vi "Fpga-6592-Top-Level.vi"() -> ()   [LabVIEW 2017]
uses:
  <vilib>/Platform/TimedLoop/XDataNode/timing_clust.ctl
  <vilib>/Platform/TimedLoop/XDataNode/nitl_modes.ctl
  <vilib>/Platform/TimedLoop/XDataNode/wakeup.ctl
  <vilib>/rvi/Emulation/niFpgaSctlEmulationGetInTimedLoop.vi
  <vilib>/rvi/Emulation/niFpgaEmulationReportErrorSimple.vi
  <vilib>/rvi/Emulation/niFpgaGetClockAttributes.vi
  <vilib>/rvi/Emulation/niFpgaCriticalErrorInLSC.vi
  <vilib>/rvi/eio/common/nirviEmuTemplateMethod_errors.vi
  <vilib>/rvi/interface/RandomDataEmulation/niFpgaRandomDataHandleErrors.vi
  <vilib>/Platform/TimedLoop/XDataNode/XDataNode.xnode
  <vilib>/eio/EIONode/EIONode.xnode
  <vilib>/rvi/DataTransferAndStorage/Container/XNode/niFpgaContainer.xnode
  <vilib>/rvi/interface/RandomDataEmulation/nirviRandomDataFpgaReadWriteTemplate.vi
  <vilib>/Platform/TimedLoop/XDataNode/XDNodeRunTimeDep.lvlib
panel:
  out "BUS_address":u32
  out "write_data":u32
  out "addr_strobe_count":u16
  out "write_strobe_count":u16
  out "read_strobe_count":u16
  in  "d_mcs_i\\IO_BUS_read_data":u32
  in  "Pulse":bool
  in  "d_mcs_i\\INTC_Interrupt":fxp<+,4,4>
  out "d_mcs_i\\gpio3_rtl_tri_o":u32
  in  "Write Interrupt":bool
  out "d_mcs_i\\gpio2_rtl_tri_o":u32
  out "d_mcs_i\\gpio1_rtl_tri_o":u32
  in  "d_mcs_i\\gpio_rtl_tri_i":u32
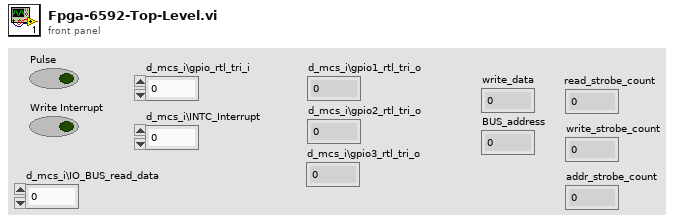
[diagram p1: front panel]
types:
  T1 = typedef "XDNodeRunTimeDep.lvlib/timing_clust.ctl" = cluster{"Expected End [f-1]":u64, "Actual End [f-1]":u64, "Finished Late? [f-1]":bool, "Expected End [i-1]":u64, "Actual End [i-1]":u64, "Finished Late? [i-1]":bool, "Expected Start [i]":u64, "Actual Start [i]":u64, "Expected Start [f]":u64, "Actual Start [f]":u64, "Source Name":string, "Structure Name":string, "Period":i64, "Deadline":i64, "Offset":i64, "Start":i64, "Priority":i32, "Timeout":i32, "Mode":T2, "Wakeup Reason":T3, "Error":errorcluster, "Source Type":string, "Secondary Source Type":string, "Global End Time":u64, "Global Start Time":u64, "Frame Duration":u64, "Iteration Duration":u64, "Assigned CPU":i32, "I/O Scan Engine Mode":u32}
  T2 = typedef "XDNodeRunTimeDep.lvlib/nitl_modes.ctl" = enum32{"No Change", "Process missed periods, maintain original phase", "Discard missed periods, maintain original phase", "Process missed periods, ignore original phase", "Discard missed periods, ignore original phase"}
  T3 = typedef "XDNodeRunTimeDep.lvlib/wakeup.ctl" = enum32{"Normal", "Aborted", "Asynchronous wakeup", "Timing source error", "Timed loop error", "Timeout"}
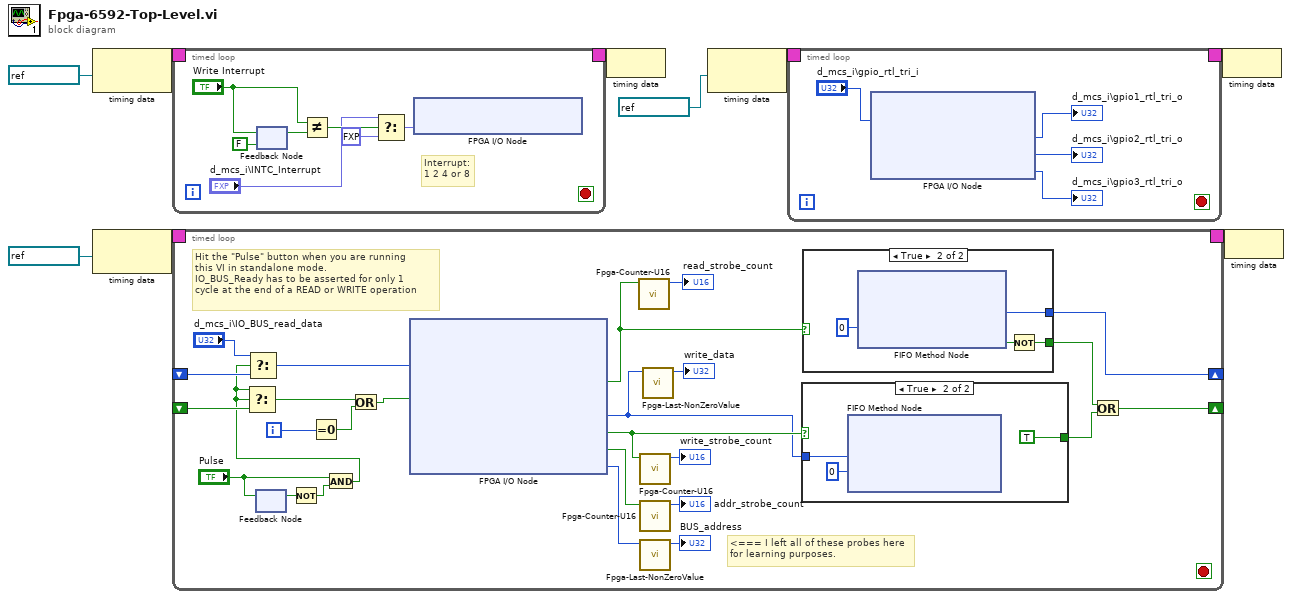
[diagram p0: block diagram]
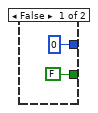
[diagram p2: hidden frame]
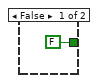
[diagram p3: hidden frame]
diagram:
  n1 = node-c288(refnum<k21> "100MHz" ("Source Name")) -> (w6:T1)
  n2 = node-c288(refnum<k21> "100MHz" ("Source Name")) -> (w9:T1)
  n3 = timed-loop {
    timing: w6 -> [_]
    timing-out: [_] -> w5
    stop <- _ stop-if-true
    # "Interrupt:\n1 2 4 or 8"
    n4 = feedback-in #1("Write Interrupt") -> ()
    n5 = feedback #1(FALSE ("Write Interrupt")) -> (w16:bool)
    n6 = Not Equal?(x="Write Interrupt", y=w16) -> (x != y?=w13:bool)
    n7 = Select(t="d_mcs_i\\INTC_Interrupt", s=w13, f=fxp<+,4,4> 0.0) -> (s? t:f=w11:fxp<+,4,4>)
    n8 = xnode "FPGA I/O Node"("d_mcs_i\\INTC_Interrupt"=w11) -> ()  [unwired: 1 in, 1 out]
  }
  n9 = timed-loop {
    timing: w9 -> [_]
    timing-out: [_] -> w8
    shift-right: [w34] -> _
    shift-left: _ -> [w38]
    shift-right: [w42] -> _
    shift-left: _ -> [w36]
    i -> [w33]
    stop <- _ stop-if-true
    # "Hit the \"Pulse\" button when you are running\nthis VI in standalone mode.\nIO_BUS_Ready has to be asserted for only 1\ncycle at the end of a READ or WRITE operation"
    # "<=== I left all of these probes here\nfor learning purposes."
    n10 = feedback #2() -> (w41:bool)  [unwired: 1 in]
    n11 = feedback-in #2("Pulse") -> ()
    n12 = Not(x=w41) -> (.not. x?=w40:bool)
    n13 = Equal To 0?(x=w33) -> (x = 0?=w19:bool)
    n14 = And(x="Pulse", y=w40) -> (x .and. y?=w22:bool)
    n15 = Select(t=w22, s=w22, f=w38) -> (s? t:f=w21:bool)
    n16 = Select(t="d_mcs_i\\IO_BUS_read_data", s=w22, f=w36) -> (s? t:f=w35:u32)
    n17 = Or(x=w21, y=w19) -> (x .or. y?=w20:bool)
    n18 = xnode "FPGA I/O Node"("d_mcs_i\\IO_BUS_read_data"=w35, "d_mcs_i\\IO_BUS_ready"=w20) -> ("d_mcs_i\\IO_BUS_read_strobe"=w31:bool, "d_mcs_i\\IO_BUS_write_data"=w26:u32, "d_mcs_i\\IO_BUS_write_strobe"=w30:bool, "d_mcs_i\\IO_BUS_addr_strobe"=w27:bool, "d_mcs_i\\IO_BUS_address"=w23:u32)  [unwired: 8 in, 9 out]
    n19 = call "Fpga-Counter-U16.vi"("d_mcs_i\\IO_BUS_read_strobe"=w31) -> ("Numeric"=→"read_strobe_count":u16)  [unwired: 10 in]
    n20 = call "Fpga-Counter-U16.vi"("d_mcs_i\\IO_BUS_read_strobe"=w30) -> ("Numeric"=→"write_strobe_count":u16)  [unwired: 10 in]
    n21 = call "Fpga-Counter-U16.vi"("d_mcs_i\\IO_BUS_read_strobe"=w27) -> ("Numeric"=→"addr_strobe_count":u16)  [unwired: 10 in]
    n22 = call "Fpga-Last-NonZeroValue.vi"("d_mcs_i\\IO_BUS_write_data in"=w23) -> ("d_mcs_i\\IO_BUS_write_data out"=→"BUS_address":u32)  [unwired: 10 in]
    n23 = call "Fpga-Last-NonZeroValue.vi"("d_mcs_i\\IO_BUS_write_data in"=w26) -> ("d_mcs_i\\IO_BUS_write_data out"=→"write_data":u32)  [unwired: 10 in]
    n24 = case shown="True" w30 {
      tunnel: w26 -> [_ w53]
      tunnel: [FALSE TRUE] -> w44
      frame False {
      }
      frame True {
        n25 = xnode ("FIFO Method Node")("Element"=w53, "Timeout"=0) -> ()  [unwired: 1 in, 2 out]
      }
    }
    n26 = case shown="True" w31 {
      tunnel: [FALSE w47] -> w43
      tunnel: [u32 0 ("Element") w48] -> w42
      frame False {
      }
      frame True {
        n27 = xnode ("FIFO Method Node")("Timeout"=0) -> ("Element"=w48:u32, "Timed Out?"=w49:bool)  [unwired: 1 in, 1 out]
        n28 = Not(x=w49) -> (.not. x?=w47:bool)
      }
    }
    n29 = Or(x=w43, y=w44) -> (x .or. y?=w34:bool)
  }
  n30 = node-c288(w5) -> ()
  n31 = node-c288(refnum<k21> "100MHz" ("Source Name")) -> (w3:T1)
  n32 = timed-loop {
    timing: w3 -> [_]
    timing-out: [_] -> w2
    stop <- _ stop-if-true
    n33 = xnode "FPGA I/O Node"("d_mcs_i\\gpio1_rtl_tri_i"="d_mcs_i\\gpio_rtl_tri_i") -> ("d_mcs_i\\gpio1_rtl_tri_o"=→"d_mcs_i\\gpio1_rtl_tri_o":u32, "d_mcs_i\\gpio2_rtl_tri_o"=→"d_mcs_i\\gpio2_rtl_tri_o":u32, "d_mcs_i\\gpio3_rtl_tri_o"=→"d_mcs_i\\gpio3_rtl_tri_o":u32)  [unwired: 4 in, 4 out]
  }
  n34 = node-c288(w2) -> ()
  n35 = node-c288(w8) -> ()
